vi "test_Expected Response Trigger - Complex-E1.vi"(8 "error in (no error)":errorcluster, 11 "TestCase in":refnum<class "Expected Response Trigger test.lvclass">) -> (0 "error out":errorcluster, 3 "TestCase out":refnum<class "Expected Response Trigger test.lvclass">)   [LabVIEW 2017, in "Expected Response Trigger test.lvclass"]
uses:
  Expected Response Trigger test.lvclass
  Libraries/SSH/Expected Response String Config.ctl
  Libraries/SSH/Search Start Point.ctl
  <vilib>/addons/_JKI Toolkits/VI Tester/TestCase.llb/TestCase.lvclass
  Libraries/SSH/SSH.lvlib
  C:/Program Files (x86)/National Instruments/LabVIEW 2017/vi.lib/addons/_JKI Toolkits/VI Tester/TestCase.llb/TestCase.lvclass
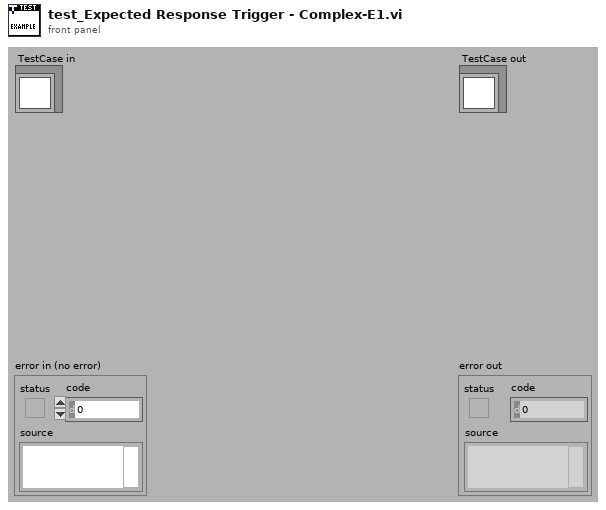
[diagram p1: front panel]
types:
  T1 = typedef "SSH.lvlib/Expected Response String Config.ctl" = cluster{"Expected Response":string, "Search Start Point":T2, "Instance Count":i32}
  T2 = typedef "SSH.lvlib/Search Start Point.ctl" = enum16{"From Start", "From End"}
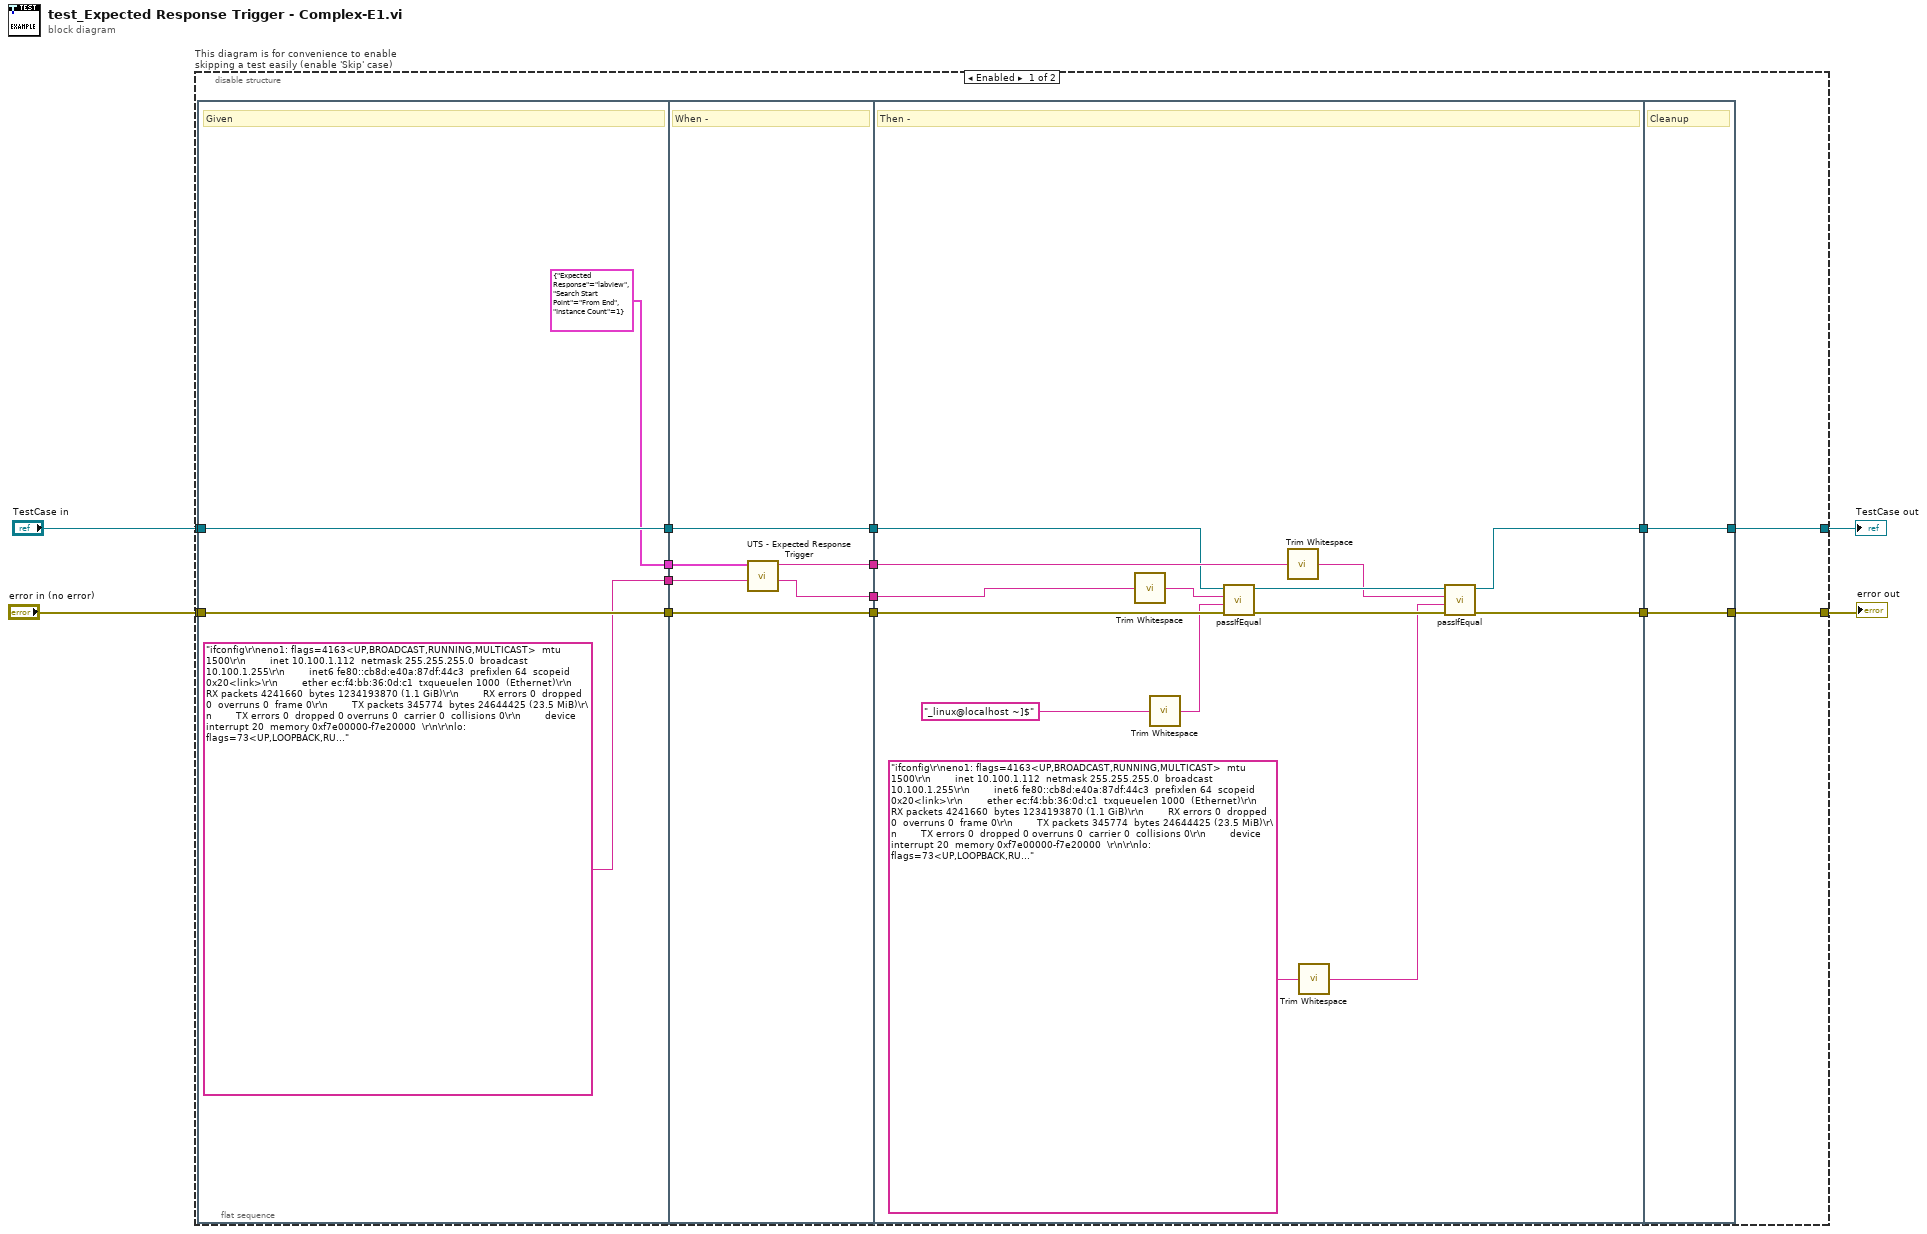
[diagram p0: block diagram]
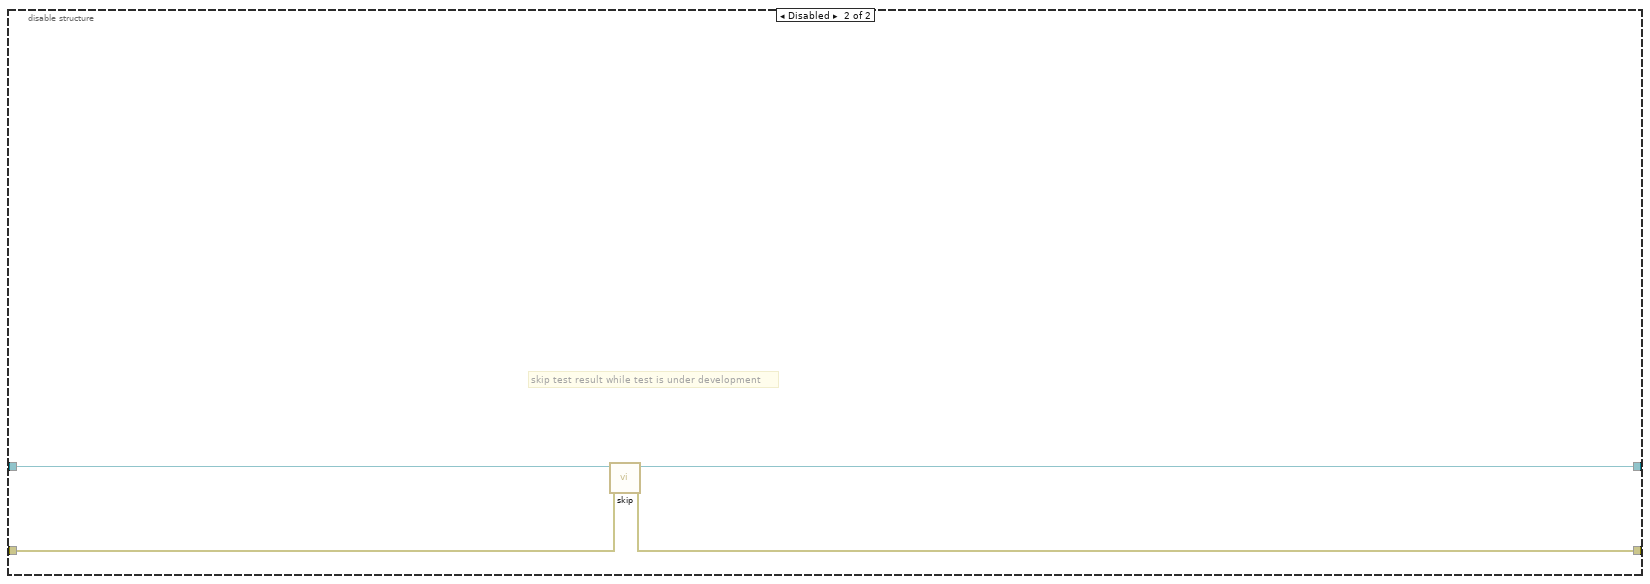
[diagram p2: hidden frame]
diagram:
  n1 = disable-structure "This diagram is for convenience to enable skipping a test easily (enable 'Skip' case)" shown="Enabled" {
    disable-tunnel: "TestCase in" -> [w11 w48]
    disable-tunnel: [w10 w46] -> w1
    disable-tunnel: [w9 w47] -> w3
    disable-tunnel: "error in (no error)" -> [w12 w45]
    frame Enabled {
      n2 = flat-sequence {
        tunnel: w12 -> [w21]
        tunnel: w11 -> [w22]
        tunnel: [w22] -> w18
        tunnel: [w21] -> w17
        tunnel: ["ifconfig\r\neno1: flags=4163<UP,BROADCAST,RUNNING,MULTICAST>  mtu 1500\r\n        inet 10.100.1.112  netmask 255.255.255.0  broadcast 10.100.1.255\r\n        inet6 fe80::cb8d:e40a:87df:44c3  prefixlen 64  scopeid 0x20<link>\r\n        ether ec:f4:bb:36:0d:c1  txqueuelen 1000  (Ethernet)\r\n        RX packets 4241660  bytes 1234193870 (1.1 GiB)\r\n        RX errors 0  dropped 0  overruns 0  frame 0\r\n        TX packets 345774  bytes 24644425 (23.5 MiB)\r\n        TX errors 0  dropped 0 overruns 0  carrier 0  collisions 0\r\n        device interrupt 20  memory 0xf7e00000-f7e20000  \r\n\r\nlo: flags=73<UP,LOOPBACK,RUNNING>  mtu 65536\r\n        inet 127.0.0.1  netmask 255.0.0.0\r\n        inet6 ::1  prefixlen 128  scopeid 0x10<host>\r\n        loop  txqueuelen 1000  (Local Loopback)\r\n        RX packets 61200  bytes 5648872 (5.3 MiB)\r\n        RX errors 0  dropped 0  overruns 0  frame 0\r\n        TX packets 61200  bytes 5648872 (5.3 MiB)\r\n        TX errors 0  dropped 0 overruns 0  carrier 0  collisions 0\r\n\r\nvirbr0: flags=4099<UP,BROADCAST,MULTICAST>  mtu 1500\r\n        inet 192.168.122.1  netmask 255.255.255.0  broadcast 192.168.122.255\r\n        ether 52:54:00:15:06:70  txqueuelen 1000  (Ethernet)\r\n        RX packets 0  bytes 0 (0.0 B)\r\n        RX errors 0  dropped 0  overruns 0  frame 0\r\n        TX packets 0  bytes 0 (0.0 B)\r\n        TX errors 0  dropped 0 overruns 0  carrier 0  collisions 0\r\n\r\n[labview_linux@localhost ~]$ \r\n[labview_linux@localhost ~]$ " ("String Buffer in")] -> w8
        tunnel: [T1 {"Expected Response"="labview", "Search Start Point"=enum."From End", "Instance Count"=1} ("Expected Response String")] -> w5
        tunnel: [w28] -> w16
        tunnel: [w27] -> w15
        tunnel: w18 -> [w28]
        tunnel: w17 -> [w27]
        tunnel: w8 -> [w26]
        tunnel: [w25] -> w7
        tunnel: [w24] -> w6
        tunnel: w5 -> [w23]
        tunnel: [w42] -> w14
        tunnel: [w31] -> w13
        tunnel: w16 -> [w40]
        tunnel: w15 -> [w38]
        tunnel: w7 -> [w41]
        tunnel: w6 -> [w39]
        tunnel: [w43] -> w9
        tunnel: [w44] -> w10
        tunnel: w14 -> [w44]
        tunnel: w13 -> [w43]
        frame #0 {
          # "Given"
        }
        frame #1 {
          # "When -"
          n3 = call "UTS - Expected Response Trigger.vi"("String Buffer in"=w26, "Expected Response"=w23) -> ("String Buffer out"=w24:string, "Response"=w25:string)  [unwired: 7 in, 1 out]
        }
        frame #2 {
          # "Then -"
          n4 = call <vilib>:"Trim Whitespace.vi"("string"=w39) -> ("trimmed string"=w35:string)  [unwired: 1 in]
          n5 = call <vilib>:"Trim Whitespace.vi"("string"="_linux@localhost ~]$" ("String Buffer in")) -> ("trimmed string"=w29:string)  [unwired: 1 in]
          n6 = call-dynamic "passIfEqual.vi"("error in (no error)"=w38, "y"=w29, "x"=w35, "TestCase in"=w40) -> ("error out"=w37:errorcluster, "TestCase out"=w36:refnum<class "Expected Response Trigger test.lvclass">)  [unwired: 6 in]
          n7 = call <vilib>:"Trim Whitespace.vi"("string"=w41) -> ("trimmed string"=w34:string)  [unwired: 1 in]
          n8 = call <vilib>:"Trim Whitespace.vi"("string"="ifconfig\r\neno1: flags=4163<UP,BROADCAST,RUNNING,MULTICAST>  mtu 1500\r\n        inet 10.100.1.112  netmask 255.255.255.0  broadcast 10.100.1.255\r\n        inet6 fe80::cb8d:e40a:87df:44c3  prefixlen 64  scopeid 0x20<link>\r\n        ether ec:f4:bb:36:0d:c1  txqueuelen 1000  (Ethernet)\r\n        RX packets 4241660  bytes 1234193870 (1.1 GiB)\r\n        RX errors 0  dropped 0  overruns 0  frame 0\r\n        TX packets 345774  bytes 24644425 (23.5 MiB)\r\n        TX errors 0  dropped 0 overruns 0  carrier 0  collisions 0\r\n        device interrupt 20  memory 0xf7e00000-f7e20000  \r\n\r\nlo: flags=73<UP,LOOPBACK,RUNNING>  mtu 65536\r\n        inet 127.0.0.1  netmask 255.0.0.0\r\n        inet6 ::1  prefixlen 128  scopeid 0x10<host>\r\n        loop  txqueuelen 1000  (Local Loopback)\r\n        RX packets 61200  bytes 5648872 (5.3 MiB)\r\n        RX errors 0  dropped 0  overruns 0  frame 0\r\n        TX packets 61200  bytes 5648872 (5.3 MiB)\r\n        TX errors 0  dropped 0 overruns 0  carrier 0  collisions 0\r\n\r\nvirbr0: flags=4099<UP,BROADCAST,MULTICAST>  mtu 1500\r\n        inet 192.168.122.1  netmask 255.255.255.0  broadcast 192.168.122.255\r\n        ether 52:54:00:15:06:70  txqueuelen 1000  (Ethernet)\r\n        RX packets 0  bytes 0 (0.0 B)\r\n        RX errors 0  dropped 0  overruns 0  frame 0\r\n        TX packets 0  bytes 0 (0.0 B)\r\n        TX errors 0  dropped 0 overruns 0  carrier 0  collisions 0\r\n\r\n[labview_linux@localhost ~]$ \r\n[labview" ("String Buffer in")) -> ("trimmed string"=w30:string)  [unwired: 1 in]
          n9 = call-dynamic "passIfEqual.vi"("error in (no error)"=w37, "y"=w30, "x"=w34, "TestCase in"=w36) -> ("error out"=w31:errorcluster, "TestCase out"=w42:refnum<class "Expected Response Trigger test.lvclass">)  [unwired: 6 in]
        }
        frame #3 {
          # "Cleanup"
        }
      }
    }
    frame Disabled {
      # "skip test result while test is under development"
      n10 = call <vilib>:"skip.vi"("error in (no error)"=w45, "TestCase in"=w48) -> ("error out"=w47:errorcluster, "TestCase out"=w46:refnum<class "Expected Response Trigger test.lvclass">)  [unwired: 8 in]
    }
  }
  "error out" <- w3
  "TestCase out" <- w1
